vi "RedistributeArmAbsolutePoseVariable.vi"(1 "DesiredPointSpacing":dbl[](array[numeric]), 2 "PathIn":T1[](array[typedef]), 3 "IndexedPathLength":dbl[](array[numeric])) -> (0 "PathOut":T1[](array[typedef]))   [LabVIEW 2018]
uses:
  TypeDefs/ArmAbsolutePosition.ctl
  ArgosLib/ArgosLib.lvlib
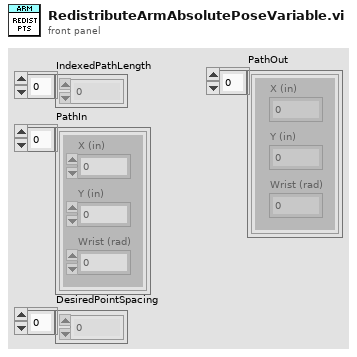
[diagram p1: front panel]
types:
  T1 = typedef "ArmAbsolutePosition.ctl" = cluster{"X (in)":dbl, "Y (in)":dbl, "Wrist (rad)":dbl}
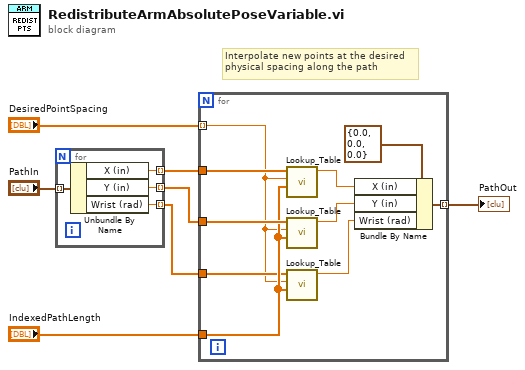
[diagram p0: block diagram]
diagram:
  # "Interpolate new points at the desired\nphysical spacing along the path"
  n1 = for {
    tunnel: "PathIn" -> [w11] mode=indexing
    tunnel: [w10] -> w5 mode=indexing
    tunnel: [w9] -> w4 mode=indexing
    tunnel: [w8] -> w1 mode=indexing
    n2 = Unbundle By Name(w11) -> ("X (in)"=w10:dbl, "Y (in)"=w9:dbl, "Wrist (rad)"=w8:dbl)
  }
  n3 = for {
    tunnel: w5 -> [w21]
    tunnel: w4 -> [w20]
    tunnel: "IndexedPathLength" -> [w15]
    tunnel: [w16] -> w3 mode=indexing
    tunnel: "DesiredPointSpacing" -> [w13] mode=indexing
    tunnel: w1 -> [w14]
    n4 = call "Lookup_Table.vi"("Y_Array"=w21, "x_in"=w13, "X_Array"=w15) -> ("y_out"=w18:dbl)  [unwired: 6 in]
    n5 = call "Lookup_Table.vi"("Y_Array"=w20, "x_in"=w13, "X_Array"=w15) -> ("y_out"=w17:dbl)  [unwired: 6 in]
    n6 = call "Lookup_Table.vi"("Y_Array"=w14, "x_in"=w13, "X_Array"=w15) -> ("y_out"=w12:dbl)  [unwired: 6 in]
    n7 = Bundle By Name(cluster=T1 {"X (in)"=0.0, "Y (in)"=0.0, "Wrist (rad)"=0.0} ("ArmAbsolutePose"), "X (in)"=w18, "Y (in)"=w17, "Wrist (rad)"=w12) -> (w16:T1)
  }
  "PathOut" <- w3
